vi "ConvertToPolarVector.vi"(8 "error in (no error)":errorcluster, 11 "CartesianVector in":refnum<class "CartesianVector.lvclass">) -> (0 "error out":errorcluster, 3 "PolarVector.lvclass":refnum<class "PolarVector.lvclass">)   [LabVIEW 2011, in "CartesianVector.lvclass"]
uses:
  CartesianVector.lvclass
  PolarVector/PolarVector.lvclass
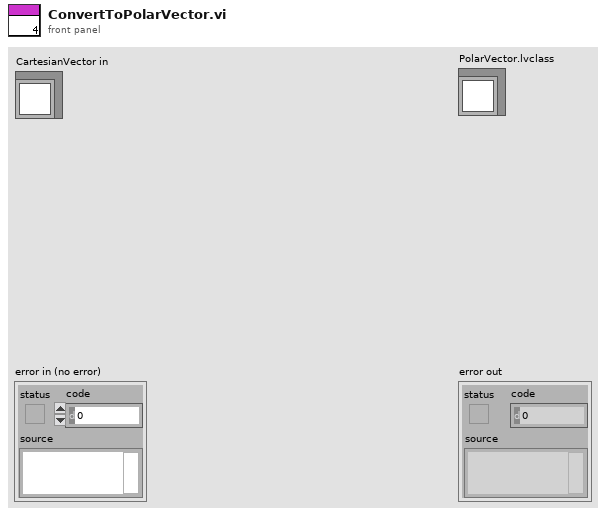
[diagram p1: front panel]
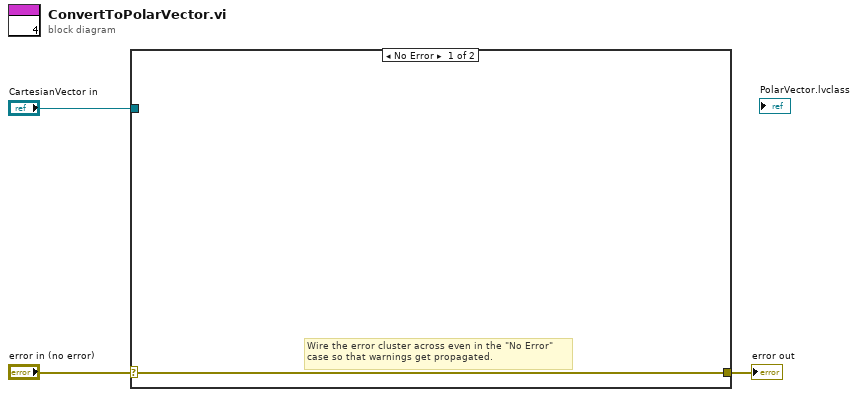
[diagram p0: block diagram]
diagram:
  n1 = case shown="No Error" "error in (no error)" {
    selector: "error in (no error)" -> [w4 w5]
    tunnel: [w4 w5] -> w2
    tunnel: "CartesianVector in" -> [_ _]
    frame No Error {
      # "Wire the error cluster across even in the \"No Error\"\ncase so that warnings get propagated."
    }
    frame Error {
    }
  }
  "error out" <- w2
